vi "Write TDATA Core.vi"(10 "raw data":bool[](array[boolean]), 11 "niInstr AXI4-Stream Writer FXP32x1 v1 FPGA in":refnum<class "niInstr AXI4-Stream Writer FXP32x1 v1 FPGA.lvclass">) -> (3 "niInstr AXI4-Stream Writer FXP32x1 v1 FPGA out":refnum<class "niInstr AXI4-Stream Writer FXP32x1 v1 FPGA.lvclass">)   [LabVIEW 2015, in "niInstr AXI4-Stream Writer FXP32x1 v1 FPGA.lvclass"]
uses:
  <instrlib>/_niInstr/CLIP Adapters/v1/FPGA/AXI4-Stream/Writer FXP32x1/niInstr AXI4-Stream Writer FXP32x1 v1 FPGA.lvclass
  <instrlib>/_niInstr/CLIP Adapters/v1/FPGA/AXI4-Stream/Writer FXP32x1/niInstr AXI4-Stream Writer FXP32x1 v1 FPGA.lvclass/niInstr AXI4-Stream Writer FXP32x1 v1 FPGA.ctl
  <vilib>/rvi/eio/common/nirviEmuTemplateMethod_errors.vi
  <instrlib>/_niInstr/Data Formatting/v1/FPGA/Private/Convert/Boolean Array to U32 Array.vi
  <vilib>/eio/EIONode/EIONode.xnode
  <instrlib>/_niInstr/Data Formatting/v1/FPGA/niInstr Data Formatting v1 FPGA.lvlib
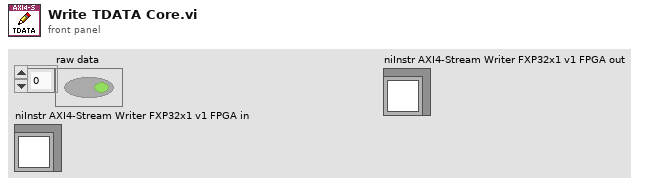
[diagram p1: front panel]
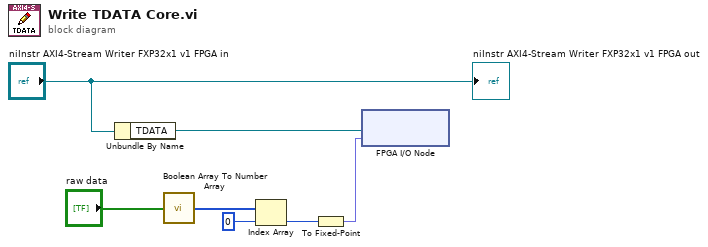
[diagram p0: block diagram]
diagram:
  n1 = Unbundle By Name("niInstr AXI4-Stream Writer FXP32x1 v1 FPGA in") -> ("TDATA"=w2:refnum<k21>)
  n2 = call-poly <instrlib>:"Boolean Array To Number Array.vi"("data in"="raw data") -> ("data out"=w6:u32[])  [unwired: 14 in]
  n3 = Index Array(array=w6, index=0) -> (element=w5:u32)
  n4 = To Fixed-Point(number=w5) -> (fixed-point=w1:fxp<+,32,32>)  [unwired: 1 in]
  n5 = xnode "FPGA I/O Node"("I/O Item"=w1, "FPGA I/O In"=w2) -> ()  [unwired: 1 out]
  "niInstr AXI4-Stream Writer FXP32x1 v1 FPGA out" <- "niInstr AXI4-Stream Writer FXP32x1 v1 FPGA in"
